vi "Overlay Image Elements.vi"(7 "Image In":T1, 8 "Error In":errorcluster) -> (0 "Error Out":errorcluster, 5 "Overlayed Image":T1(plugin-control))   [LabVIEW 2018]
uses:
  <vilib>/vision/Image Controls.llb/IMAQ Image.ctl
  Table Data.vi
  Red Team Data.vi
  Blue Team Data.vi
  Ball Data.vi
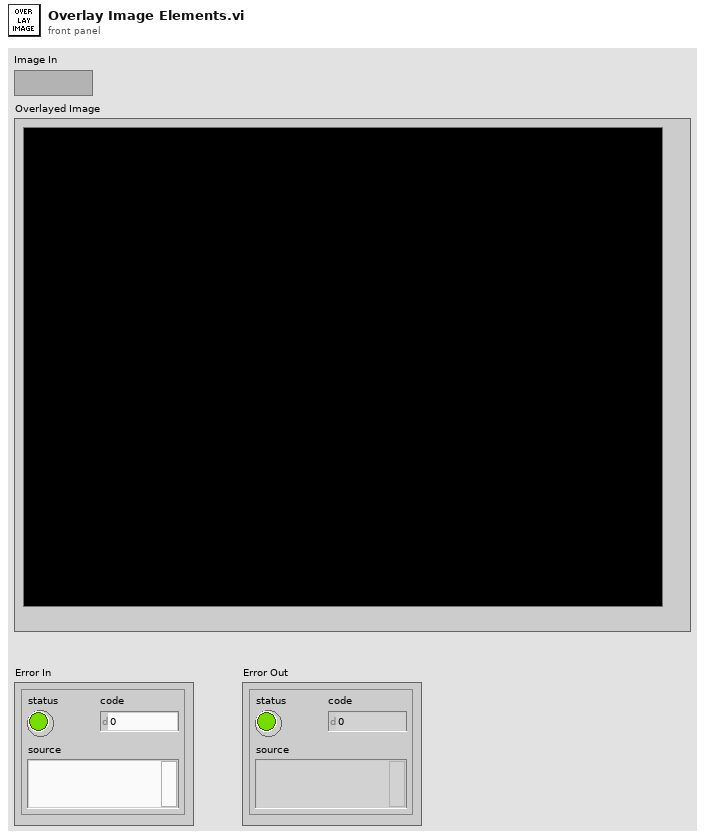
[diagram p1: front panel]
types:
  T1 = typedef "IMAQ Image.ctl" = refnum<image>
  T2 = cluster{"Object Center":cluster{"X":sgl, "Y":sgl}, "Bounding Box":cluster{"X Left":i32, "Y Top":i32, "X Right":i32, "Y Bottom":i32}, "Area":sgl, "Orientation":sgl, "Aspect Ratio":sgl, "Nb Holes":i32}
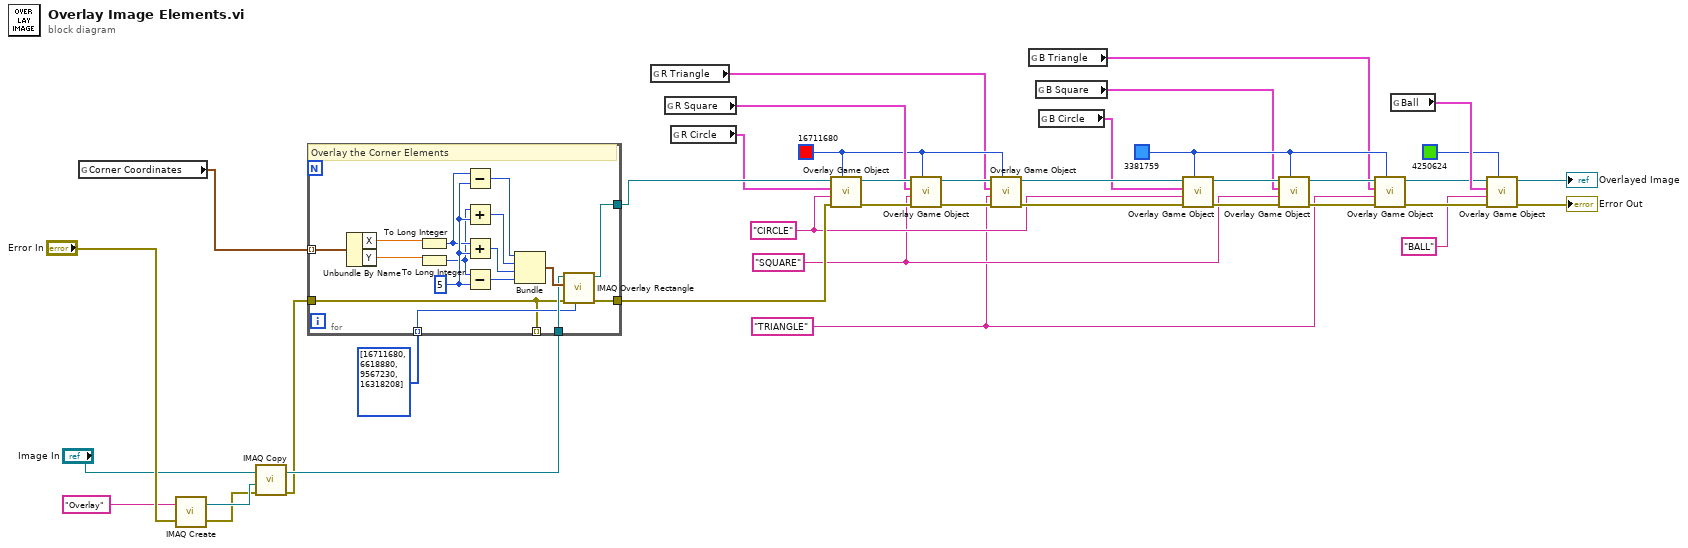
[diagram p0: block diagram]
diagram:
  w21 = u32 3381759 ("Color")
  w15 = "TRIANGLE" ("Name")
  w16 = "SQUARE" ("Name")
  w29 = u32 16711680 ("Color")
  w17 = "CIRCLE" ("Name")
  n1 = global read "Table Data.vi" "Corner Coordinates"() -> (w38:cluster{"X":sgl, "Y":sgl}[])
  n2 = call "IMAQ Create"("Image Name"="Overlay", "error in (no error)"="Error In") -> ("New Image"=w5:T1, "error out"=w4:errorcluster)  [unwired: 3 in]
  n3 = call "IMAQ Copy"("error in (no error)"=w4, "Image Dst"=w5, "Image Src"="Image In") -> ("error out"=w1:errorcluster, "Image Dst Out"=w2:T1)  [unwired: 3 in]
  n4 = for {
    tunnel: [w47] -> w36
    tunnel: w38 -> [w45] mode=indexing
    tunnel: [w46] -> w37
    tunnel: w2 -> [w42]
    tunnel: [w40] -> _ mode=indexing
    tunnel: u32[] [16711680, 6618880, 9567230, 16318208] -> [w41] mode=indexing
    tunnel: w1 -> [w40]
    w55 = 5
    # "Overlay the Corner Elements"
    n5 = Unbundle By Name(w45) -> ("X"=w44:sgl, "Y"=w43:sgl)
    n6 = To Long Integer(number=w44) -> (32bit integer=w54:i32)
    n7 = To Long Integer(number=w43) -> (32bit integer=w53:i32)
    n8 = Subtract(x=w54, y=w55) -> (x-y=w52:i32)
    n9 = Add(x=w53, y=w55) -> (x+y=w51:i32)
    n10 = Add(x=w54, y=w55) -> (x+y=w50:i32)
    n11 = Subtract(x=w53, y=w55) -> (x-y=w49:i32)
    n12 = Bundle(w52, w51, w50, w49) -> (w48:cluster{i32, i32, i32, i32})  [unwired: 1 in]
    n13 = call "IMAQ Overlay Rectangle"("Color"=w41, "error in (no error)"=w40, "Rectangle"=w48, "Image"=w42) -> ("error out"=w47:errorcluster, "Image Out"=w46:T1)  [unwired: 6 in]
  }
  n14 = global read "Red Team Data.vi" "R Triangle"() -> (w28:T2)
  n15 = global read "Red Team Data.vi" "R Square"() -> (w32:T2)
  n16 = global read "Red Team Data.vi" "R Circle"() -> (w35:T2)
  n17 = call "Overlay Game Object.vi"("Color"=w29, "error in (no error)"=w36, "Name"=w17, "Object"=w35, "Image In"=w37) -> ("error out"=w34:errorcluster, "Image Out"=w33:T1)  [unwired: 5 in]
  n18 = call "Overlay Game Object.vi"("Color"=w29, "error in (no error)"=w34, "Name"=w16, "Object"=w32, "Image In"=w33) -> ("error out"=w31:errorcluster, "Image Out"=w30:T1)  [unwired: 5 in]
  n19 = call "Overlay Game Object.vi"("Color"=w29, "error in (no error)"=w31, "Name"=w15, "Object"=w28, "Image In"=w30) -> ("error out"=w27:errorcluster, "Image Out"=w24:T1)  [unwired: 5 in]
  n20 = global read "Blue Team Data.vi" "B Triangle"() -> (w18:T2)
  n21 = global read "Blue Team Data.vi" "B Square"() -> (w19:T2)
  n22 = global read "Blue Team Data.vi" "B Circle"() -> (w20:T2)
  n23 = call "Overlay Game Object.vi"("Color"=w21, "error in (no error)"=w27, "Name"=w17, "Object"=w20, "Image In"=w24) -> ("error out"=w26:errorcluster, "Image Out"=w23:T1)  [unwired: 5 in]
  n24 = call "Overlay Game Object.vi"("Color"=w21, "error in (no error)"=w26, "Name"=w16, "Object"=w19, "Image In"=w23) -> ("error out"=w25:errorcluster, "Image Out"=w22:T1)  [unwired: 5 in]
  n25 = call "Overlay Game Object.vi"("Color"=w21, "error in (no error)"=w25, "Name"=w15, "Object"=w18, "Image In"=w22) -> ("error out"=w12:errorcluster, "Image Out"=w13:T1)  [unwired: 5 in]
  n26 = global read "Ball Data.vi" "Ball"() -> (w14:T2)
  n27 = call "Overlay Game Object.vi"("Color"=u32 4250624, "error in (no error)"=w12, "Name"="BALL", "Object"=w14, "Image In"=w13) -> ("error out"=→"Error Out":errorcluster, "Image Out"=→"Overlayed Image":T1)  [unwired: 5 in]
